vi "dvp Vi Get Soft Trigger Loop State.vi"(10 "pSoftTriggerLoopState":i32, 11 "handle":u32) -> (2 "pSoftTriggerLoopState out":i32, 3 "function return":u32(ring))   [LabVIEW 2018, in "LabViewDVPCamera.lvlib"]
doc: "LabviewDvp2Api dvpStatus dvpViGetSoftTriggerLoopState(dvpHandle handle, BOOL *pSoftTriggerLoopState);"
uses:
  LabViewDVPCamera.lvlib
  LabViewDVPCamera/LabViewDVPCamera.dll
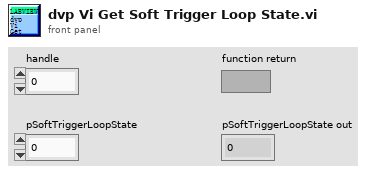
[diagram p1: front panel]
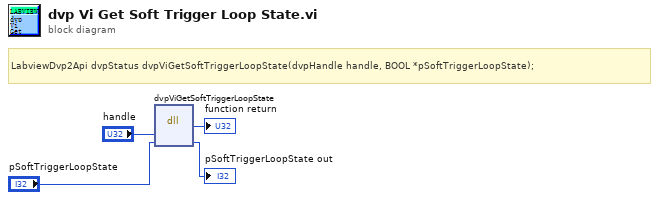
[diagram p0: block diagram]
diagram:
  # "LabviewDvp2Api dvpStatus dvpViGetSoftTriggerLoopState(dvpHandle handle, BOOL *pSoftTriggerLoopState);"
  n1 = dll-call lib="C:/Program Files (x86)/DVP2 Labview cn 64/Sample/LabViewDVPCamera/LabViewDVPCamera.*" fn="dvpViGetSoftTriggerLoopState"("handle"="handle", "pSoftTriggerLoopState"="pSoftTriggerLoopState") -> (→"function return":u32, "pSoftTriggerLoopState"=→"pSoftTriggerLoopState out":i32)  [unwired: 4 in, 2 out]
